vi "sub_edge_V1.vi"(11 "signal_in":bool) -> (1 "edge":bool, 2 "fail_edge":bool, 3 "raise_edge":bool)   [LabVIEW 2020]
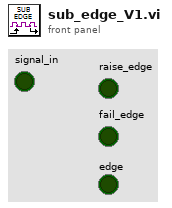
[diagram p1: front panel]
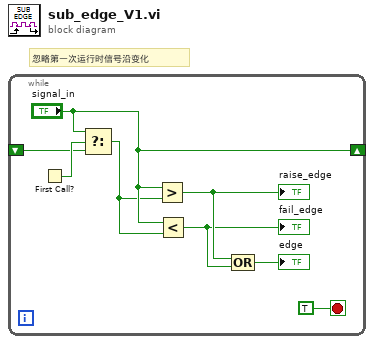
[diagram p0: block diagram]
diagram:
  # "忽略第一次运行时信号沿变化"
  n1 = while {
    shift-right: ["signal_in"] -> _
    shift-left: _ -> [w5]
    stop <- TRUE stop-if-true
    n2 = First Call?() -> (First Call?: T/F=w7:bool)
    n3 = Select(t="signal_in", s=w7, f=w5) -> (s? t:f=w4:bool)
    n4 = Greater?(x="signal_in", y=w4) -> (0:w3:bool)
    "raise_edge" <- w3
    n5 = Less?(x="signal_in", y=w4) -> (x < y?=w2:bool)
    "fail_edge" <- w2
    n6 = Compound Arithmetic op=OR(w3, w2) -> (→"edge":bool)
  }
